vi "Read String.vi"(8 "error in (no error)":errorcluster, 10 "Ctl Refnum":refnum<vi>, 11 "Worksheet Reference":refnum<k7>) -> (0 "error out":errorcluster)   [LabVIEW 2015]
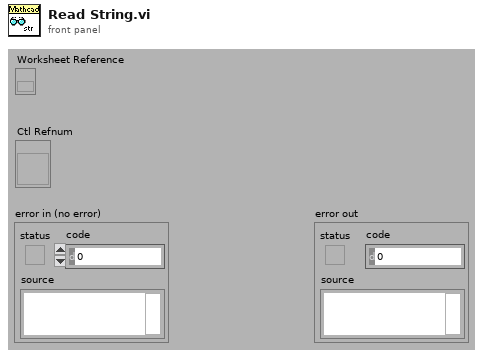
[diagram p1: front panel]
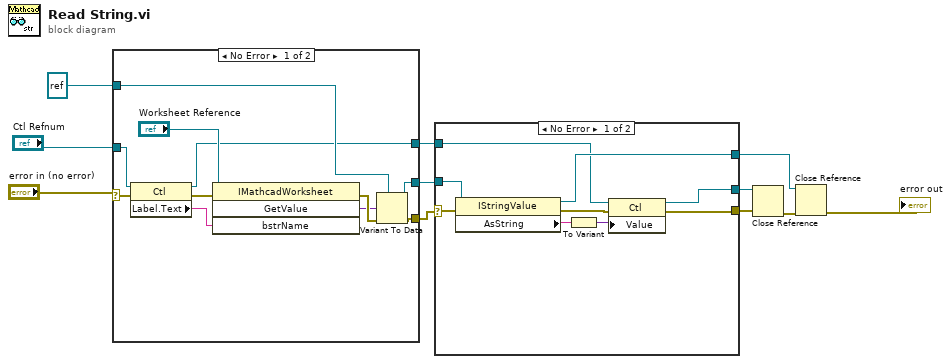
[diagram p0: block diagram]
diagram:
  n1 = case shown="No Error" "error in (no error)" {
    selector: "error in (no error)" -> [w16 w25]
    tunnel: [w22 w25] -> w10
    tunnel: refnum<k7> refnum ("Mathcad.IStringValue") -> [w18 w24]
    tunnel: [w17 w24] -> w8
    tunnel: "Ctl Refnum" -> [w14 w23]
    tunnel: [w12 w23] -> w4
    frame No Error {
      n2 = property class="Ctl"(reference=w14, error in=w16) -> (reference out=w12:refnum<vi>, error out=w15:errorcluster, "Label.Text"=w13:string)
      n3 = invoke class="IMathcadWorksheet" method="GetValue"(reference="Worksheet Reference", error in=w15, "bstrName"=w13) -> (error out=w21:errorcluster, "GetValue"=w20:variant)  [unwired: 1 in, 2 out]
      n4 = Variant To Data(error in=w21, type=w18, Variant=w20) -> (data=w17:refnum<k7>, error out=w22:errorcluster)
    }
    frame Error {
    }
  }
  n5 = case shown="No Error" w10 {
    selector: w10 -> [w33 w36]
    tunnel: [w27 w36] -> w3
    tunnel: w8 -> [w34 w37]
    tunnel: [w32 w37] -> w7
    tunnel: w4 -> [w28 w35]
    tunnel: [w26 w35] -> w1
    frame No Error {
      n6 = property class="IStringValue"(reference=w34, error in=w33) -> (reference out=w32:refnum<k7>, error out=w29:errorcluster, "AsString"=w31:string)
      n7 = To Variant(anything=w31) -> (Variant=w30:variant)
      n8 = property class="Ctl"(reference=w28, error in=w29, "Value"=w30) -> (reference out=w26:refnum<vi>, error out=w27:errorcluster)
    }
    frame Error {
    }
  }
  n9 = Close Reference(reference=w1, error in (no error)=w3) -> (error out=w2:errorcluster)
  n10 = Close Reference(reference=w7, error in (no error)=w2) -> (error out=→"error out":errorcluster)
